vi "Init.vi"(8 "Error In":errorcluster, 10 "IConfigure":refnum<class "IConfigure.lvclass">, 11 "object in":refnum<class "Scope Base.lvclass">) -> (0 "Error Out":errorcluster, 3 "object out":refnum<class "Scope Base.lvclass">)   [LabVIEW 2023, in "Scope.lvlib" / "Scope Base.lvlib" / "Scope Base.lvclass"]
uses:
  Scope Base.lvclass
  Scope Base.lvclass/Scope Base.ctl
  Interfaces/IConfigure/IConfigure.lvclass
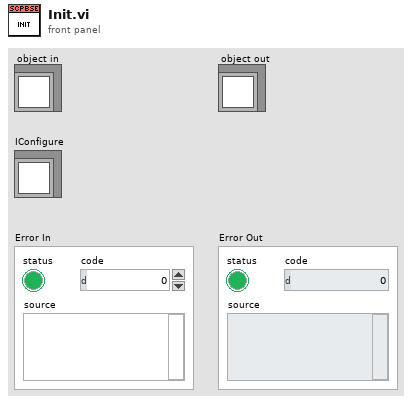
[diagram p1: front panel]
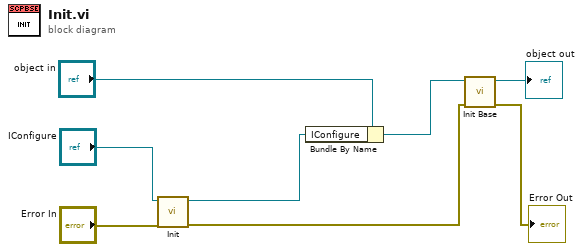
[diagram p0: block diagram]
diagram:
  n1 = call-dynamic "Init.vi"("error in"="Error In", "IConfigure in"="IConfigure") -> ("error out"=w4:errorcluster, "IConfigure out"=w7:refnum<class "IConfigure.lvclass">)  [unwired: 8 in]
  n2 = Bundle By Name(cluster="object in", "IConfigure"=w7) -> (w2:refnum<class "Scope Base.lvclass">)
  n3 = call-dynamic "Init Base.vi"("Error In"=w4, "object in"=w2) -> ("Error Out"=→"Error Out":errorcluster, "object out"=→"object out":refnum<class "Scope Base.lvclass">)  [unwired: 8 in]
